vi "Client.vi"() -> ()   [LabVIEW 2021]
uses:
  <vilib>/Utility/miscctls.llb/LVPositionTypeDef.ctl
  MessageType.ctl
panel:
  in  "Server IP Address":string="localhost"
  in  "Stop":bool
  in  "State Change":bool=TRUE
  out "Status":string
  out "GS":enum16{"Player 1 shoot", "Player 2 Shoot"}(ring)
  out "Player 2 Score":u8
  out "Player 1 Score":u8
  in  "Goal Post":cluster{"left":i16, "Size":i16}={"left"=110, "Size"=125}
  out "Goal Post":T1={"left"=110, "top"=0, "right"=235, "bottom"=15}
  out "Box":T1={"left"=139, "top"=147, "right"=181, "bottom"=180}
  out "goal?":bool=TRUE
  out "Del GK":dbl
  out "Defend":bool
  in  "GK":cluster{"horizontal":dbl, "vertical":dbl}={"horizontal"=175.0, "vertical"=20.0}
  in  "Box Size":cluster{"horizontal":dbl, "Vertical":dbl}={"horizontal"=21.0, "Vertical"=33.0}
  in  "Reset":bool
  out "del x":dbl=-0.26666666666666666
  in  "wait":u32=10
  in  "shot?":bool
  in  "Power":dbl(slide)=1.4141414141414141 scale=0.0..10.0
  in  "Ball Size":i16=9
  in  "Ball":cluster{"horizontal":dbl, "vertical":dbl}={"horizontal"=160.0, "vertical"=180.0}
  in  "Shoot":bool
  out "Ground":picture
  # "PLAYER 2"
  # "Misc. Controls"
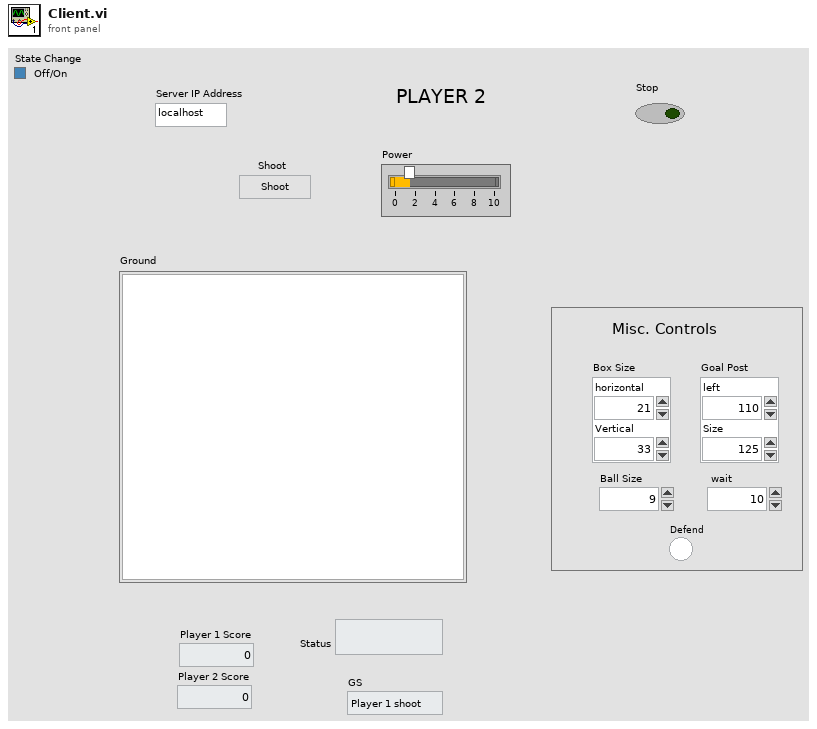
[diagram p1: front panel]
types:
  T1 = cluster{"left":i16, "top":i16, "right":i16, "bottom":i16}
  T2 = typedef "MessageType.ctl" = enum16{"Shoot", "Defend", "Reset", "Score"}
  T3 = typedef "LVPositionTypeDef.ctl" = cluster{"Left":i32, "Top":i32}
  T4 = typedef "LVPoint32TypeDef.ctl" = cluster{"Horizontal":i32, "Vertical":i32}
  T5 = typedef "eventsource.ctl" = u32
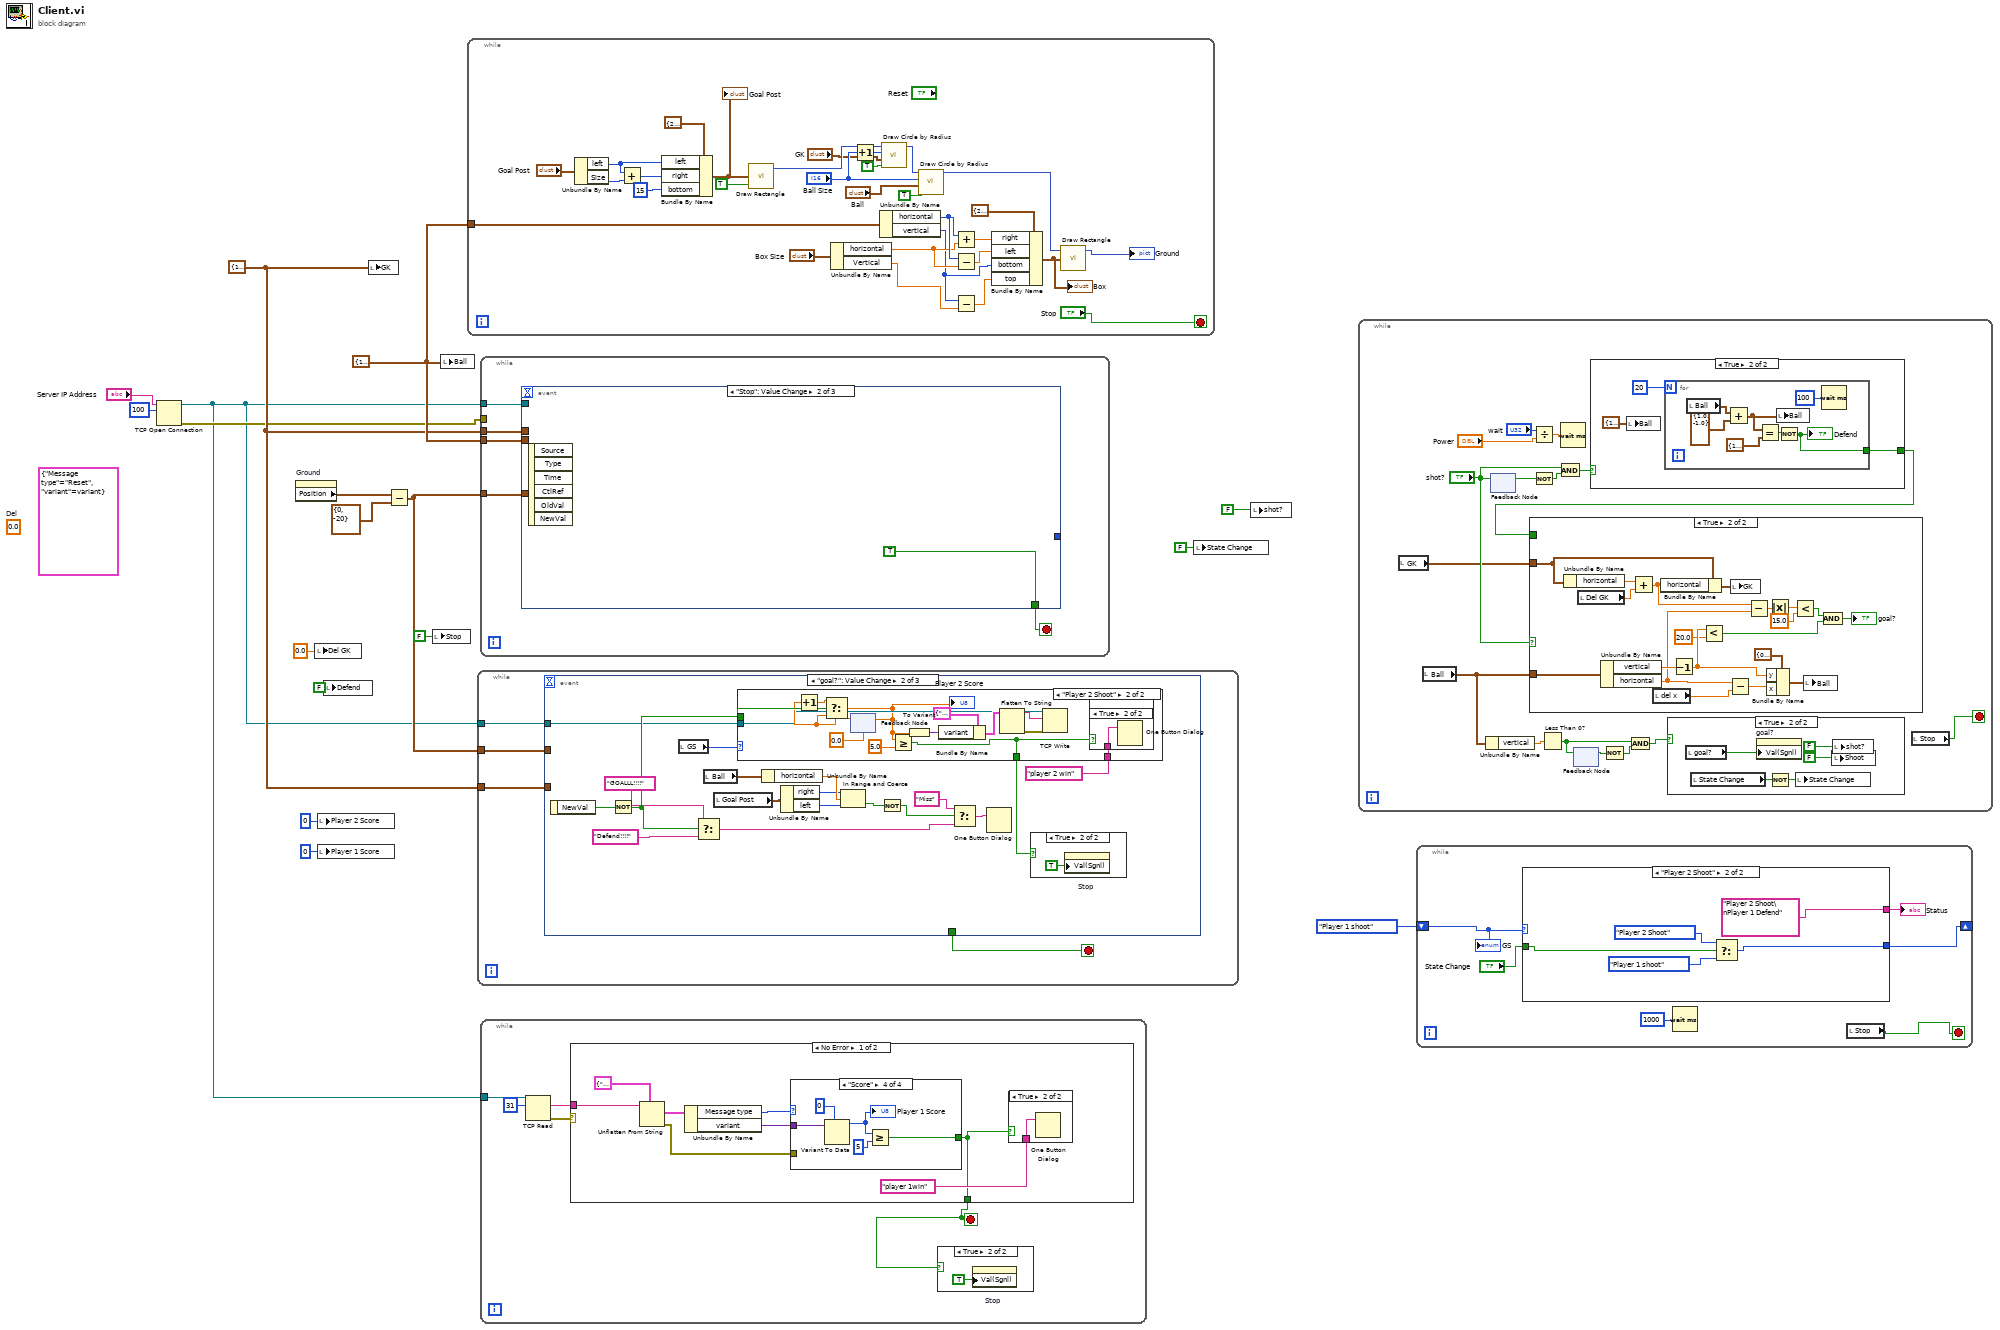
[diagram p0: block diagram]
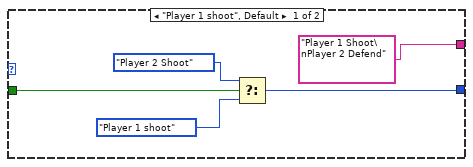
[diagram p2: hidden frame]
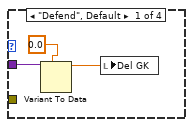
[diagram p5: hidden frame]
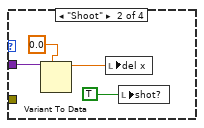
[diagram p6: hidden frame]
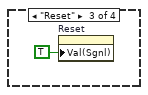
[diagram p7: hidden frame]
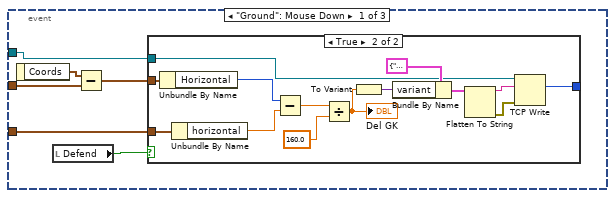
[diagram p9: hidden frame]
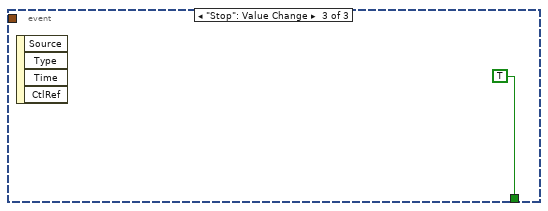
[diagram p14: hidden frame]
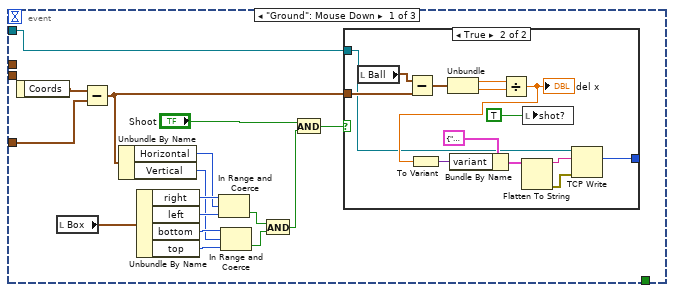
[diagram p18: hidden frame]
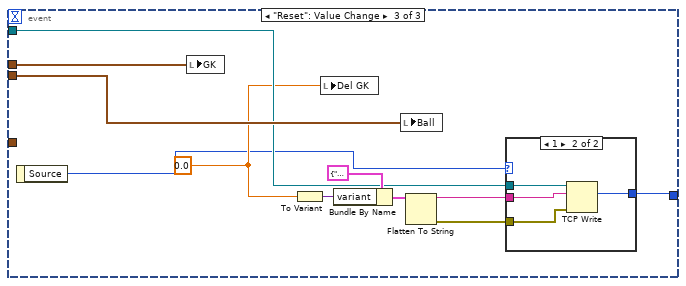
[diagram p20: hidden frame]
diagram:
  (unwired) 0.0  # Del
  (unwired) cluster{"Message type":T2, "variant":variant} {"Message type"=enum."Reset", "variant"=variant}
  w11 = cluster{"horizontal":dbl, "vertical":dbl} {"horizontal"=175.0, "vertical"=20.0} ("GK")
  w14 = cluster{"horizontal":i16, "vertical":i16} {"horizontal"=160, "vertical"=180} ("Ball")
  n1 = TCP Open Connection(address="Server IP Address", remote port or service name=u16 100 ("port")) -> (connection ID=w7:refnum<k5>, error out=w8:errorcluster)  [unwired: 3 in]
  n2 = property on="Ground" class="Pict"() -> ("Position"=w16:T3)  [unwired: 2 in, 2 out]
  n3 = local write "Del GK"(0.0 ("Del GK")) -> ()
  n4 = local write "Player 2 Score"(u8 0 ("Player 2 Score")) -> ()
  n5 = local write "Player 1 Score"(u8 0 ("Player 1 Score")) -> ()
  n6 = local write "Defend"(FALSE ("def")) -> ()
  n7 = local write "GK"(w11) -> ()
  n8 = Subtract(x=w16, y=T3 {"Left"=0, "Top"=-20}) -> (x-y=w13:T3)
  n9 = local write "Stop"(FALSE ("Stop")) -> ()
  n10 = local write "Ball"(w14) -> ()
  n11 = while {
    tunnel: w14 -> [w28]
    stop <- "Stop" stop-if-true
    n12 = Unbundle By Name("Goal Post") -> ("left"=w20:i16, "Size"=w19:i16)
    n13 = Add(x=w20, y=w19) -> (x+y=w43:i16)
    n14 = Bundle By Name(cluster=T1 {"left"=22, "top"=0, "right"=10, "bottom"=10} ("rect"), "left"=w20, "right"=w43, "bottom"=i16 15) -> (w44:T1)
    "Goal Post" <- w44
    n15 = call <vilib>:"Draw Rectangle.vi"("rect"=w44, "fill?(F)"=TRUE) -> ("new picture"=w25:picture)  [unwired: 7 in]
    n16 = Unbundle By Name("Box Size") -> ("horizontal"=w36:dbl, "Vertical"=w33:dbl)
    n17 = Increment(x="Ball Size") -> (x+1=w22:i16)
    n18 = Unbundle By Name(w28) -> ("horizontal"=w37:i16, "vertical"=w35:i16)
    n19 = call <vilib>:"Draw Circle by Radius.vi"("fill?(F)"=TRUE, "pixel center"="GK", "radius"=w22, "picture"=w25) -> ("new picture"=w23:picture)  [unwired: 7 in]
    n20 = call <vilib>:"Draw Circle by Radius.vi"("fill?(F)"=TRUE, "pixel center"="Ball", "radius"="Ball Size", "picture"=w23) -> ("new picture"=w30:picture)  [unwired: 7 in]
    n21 = Add(x=w37, y=w36) -> (x+y=w38:dbl)
    n22 = Subtract(x=w37, y=w36) -> (x-y=w34:dbl)
    n23 = Subtract(x=w35, y=w33) -> (x-y=w32:dbl)
    n24 = Bundle By Name(cluster=T1 {"left"=22, "top"=0, "right"=10, "bottom"=10} ("rect"), "right"=w38, "left"=w34, "bottom"=w35, "top"=w32) -> (w31:T1)
    "Box" <- w31
    n25 = call <vilib>:"Draw Rectangle.vi"("picture"=w30, "rect"=w31) -> ("new picture"=→"Ground":picture)  [unwired: 7 in]
  }
  n26 = while {
    tunnel: w13 -> [w51]
    tunnel: w11 -> [w50]
    tunnel: w7 -> [w49]
    stop <- w48 stop-if-true
    n27 = event shown="[1] \"goal?\": Value Change" {
      selector: _ -> [_ _ _]
      dyn-events: _ -> [_ _ _]
      timeout: _ -> [_ _ _]
      tunnel: w51 -> [w56 _ _]
      tunnel: w50 -> [w54 _ _]
      tunnel: w49 -> [w52 w75 _]
      tunnel: [_ _ TRUE] -> w48
      event "Ground": Mouse Down {
        n28 = event-data() -> ("Coords"=w57:T4)  [unwired: 1 in]
        n29 = local read "Defend"() -> (w53:bool)
        n30 = Subtract(x=w57, y=w56) -> (x-y=w55:T4)
        n31 = case shown="True" w53 {
          tunnel: w55 -> [_ w71]
          tunnel: w54 -> [_ w70]
          tunnel: w52 -> [_ w60]
          tunnel: [_ w58] -> _
          frame False {
          }
          frame True {
            n32 = Unbundle By Name(w71) -> ("Horizontal"=w69:i32)
            n33 = Unbundle By Name(w70) -> ("horizontal"=w68:dbl)
            n34 = Subtract(x=w69, y=w68) -> (x-y=w67:dbl)
            n35 = Divide(x=w67, y=160.0) -> (x/y=w59:dbl)
            "Del GK" <- w59
            n36 = To Variant(anything=w59) -> (Variant=w64:variant)
            n37 = Bundle By Name(cluster=cluster{"Message type":T2, "variant":variant} {"Message type"=enum."Defend", "variant"=variant}, "variant"=w64) -> (w63:cluster{"Message type":T2, "variant":variant})
            n38 = Flatten To String(anything=w63) -> (data string=w61:string, error out=w62:errorcluster)  [unwired: 3 in, 1 out]
            n39 = TCP Write(connection ID=w60, data in=w61, error in (no error)=w62) -> (bytes written=w58:i32)  [unwired: 1 in, 2 out]
          }
        }
      }
      event "goal?": Value Change {
        n40 = event-data() -> ("NewVal"=w89:bool)  [unwired: 1 in]
        n41 = Not(x=w89) -> (.not. x?=w76:bool)
        n42 = local read "GS"() -> (w74:enum16{"Player 1 shoot", "Player 2 Shoot"})
        n43 = Select(t="GOALLL!!!!", s=w76, f="Defend!!!!") -> (s? t:f=w78:string)
        n44 = local read "Ball"() -> (w82:cluster{"horizontal":dbl, "vertical":dbl})
        n45 = local read "Goal Post"() -> (w83:T1)
        n46 = case shown="\"Player 2 Shoot\"" w74 {
          tunnel: w76 -> [_ w99]
          tunnel: w75 -> [_ w96]
          tunnel: "player 2 win" -> [_ w94]
          tunnel: [_ w91] -> w72
          frame "Player 1 shoot", Default {
          }
          frame "Player 2 Shoot" {
            n47 = feedback #1(0.0) -> (w97:dbl)
            n48 = Increment(x=w97) -> (x+1=w98:dbl)
            n49 = Select(t=w98, s=w99, f=w97) -> (s? t:f=w93:dbl)
            "Player 2 Score" <- w93
            n50 = feedback-in #1(w93) -> ()
            n51 = Greater Or Equal?(x=w93, y=5.0) -> (x >= y?=w91:bool)
            n52 = To Variant(anything=w93) -> (Variant=w103:variant)
            n53 = Bundle By Name(cluster=cluster{"Message type":T2, "variant":variant} {"Message type"=enum."Score", "variant"=variant}, "variant"=w103) -> (w102:cluster{"Message type":T2, "variant":variant})
            n54 = Flatten To String(anything=w102) -> (data string=w100:string, error out=w101:errorcluster)  [unwired: 3 in, 1 out]
            n55 = TCP Write(connection ID=w96, data in=w100, error in (no error)=w101) -> ()  [unwired: 1 in, 3 out]
            n56 = case shown="True" w91 {
              tunnel: w94 -> [_ w105]
              frame False {
              }
              frame True {
                n57 = One Button Dialog(message=w105) -> ()  [unwired: 1 in, 1 out]
              }
            }
          }
        }
        n58 = Unbundle By Name(w82) -> ("horizontal"=w86:dbl)
        n59 = Unbundle By Name(w83) -> ("right"=w84:i16, "left"=w85:i16)
        n60 = In Range and Coerce(upper limit=w84, x=w86, lower limit=w85) -> (In Range?=w81:bool)  [unwired: 1 out]
        n61 = Not(x=w81) -> (.not. x?=w77:bool)
        n62 = Select(t="Miss", s=w77, f=w78) -> (s? t:f=w79:string)
        n63 = One Button Dialog(message=w79) -> ()  [unwired: 1 in, 1 out]
        n64 = case shown="True" w72 {
          frame False {
          }
          frame True {
            n65 = property on="Stop" class="Bool (strict)"("Val(Sgnl)"=TRUE ("Value (Signaling)")) -> ()  [unwired: 2 in, 2 out]
          }
        }
      }
      event "Stop": Value Change {
        n66 = event-data() -> ()  [unwired: 1 in, 4 out]
      }
    }
  }
  n67 = while {
    tunnel: w13 -> [w111]
    tunnel: w14 -> [w110]
    tunnel: w11 -> [w109]
    tunnel: w7 -> [w108]
    tunnel: w8 -> [_]
    stop <- w107 stop-if-true
    n68 = event shown="[1] \"Stop\": Value Change" {
      selector: _ -> [_ _ _]
      dyn-events: _ -> [_ _ _]
      timeout: _ -> [_ _ _]
      tunnel: w111 -> [w125 _ _]
      tunnel: w110 -> [_ _ w153]
      tunnel: w109 -> [_ _ w152]
      tunnel: w108 -> [w113 _ w146]
      tunnel: [_ _ w144] -> _
      tunnel: [_ TRUE _] -> w107
      event "Ground": Mouse Down {
        n69 = event-data() -> ("Coords"=w126:T4)  [unwired: 1 in]
        n70 = local read "Box"() -> (w124:T1)
        n71 = Subtract(x=w126, y=w125) -> (x-y=w119:T4)
        n72 = Unbundle By Name(w119) -> ("Horizontal"=w118:i32, "Vertical"=w117:i32)
        n73 = Unbundle By Name(w124) -> ("right"=w123:i16, "left"=w122:i16, "bottom"=w121:i16, "top"=w120:i16)
        n74 = In Range and Coerce(upper limit=w123, x=w118, lower limit=w122) -> (In Range?=w115:bool)  [unwired: 1 out]
        n75 = In Range and Coerce(upper limit=w121, x=w117, lower limit=w120) -> (In Range?=w116:bool)  [unwired: 1 out]
        n76 = And(x=w115, y=w116) -> (x .and. y?=w112:bool)
        n77 = And(x="Shoot", y=w112) -> (x .and. y?=w114:bool)
        n78 = case shown="True" w114 {
          tunnel: w119 -> [_ w140]
          tunnel: w113 -> [_ w129]
          tunnel: [_ w128] -> _
          frame False {
          }
          frame True {
            n79 = local read "Ball"() -> (w139:cluster{"horizontal":dbl, "vertical":dbl})
            n80 = Subtract(x=w139, y=w140) -> (x-y=w138:cluster{dbl, dbl})
            n81 = Unbundle(w138) -> (w137:dbl, w136:dbl)
            n82 = Divide(x=w137, y=w136) -> (x/y=w134:dbl)
            "del x" <- w134
            n83 = To Variant(anything=w134) -> (Variant=w133:variant)
            n84 = Bundle By Name(cluster=cluster{"Message type":T2, "variant":variant} {"Message type"=enum."Shoot", "variant"=variant}, "variant"=w133) -> (w132:cluster{"Message type":T2, "variant":variant})
            n85 = Flatten To String(anything=w132) -> (data string=w130:string, error out=w131:errorcluster)  [unwired: 3 in, 1 out]
            n86 = local write "shot?"(TRUE ("Checkbox")) -> ()
            n87 = TCP Write(connection ID=w129, data in=w130, error in (no error)=w131) -> (bytes written=w128:i32)  [unwired: 1 in, 2 out]
          }
        }
      }
      event "Stop": Value Change {
        n88 = event-data() -> ()  [unwired: 1 in, 6 out]
      }
      event "Reset": Value Change {
        w145 = 0.0 ("Del GK")
        n89 = event-data() -> ("Source"=w143:T5)  [unwired: 1 in]
        n90 = local write "GK"(w152) -> ()
        n91 = To Variant(anything=w145) -> (Variant=w150:variant)
        n92 = local write "Del GK"(w145) -> ()
        n93 = Bundle By Name(cluster=cluster{"Message type":T2, "variant":variant} {"Message type"=enum."Reset", "variant"=variant}, "variant"=w150) -> (w149:cluster{"Message type":T2, "variant":variant})
        n94 = local write "Ball"(w153) -> ()
        n95 = Flatten To String(anything=w149) -> (data string=w147:string, error out=w148:errorcluster)  [unwired: 3 in, 1 out]
        n96 = case shown="1" w143 {
          tunnel: w148 -> [_ w157]
          tunnel: w147 -> [_ w156]
          tunnel: w146 -> [_ w155]
          tunnel: [_ w154] -> w144
          frame 0, Default {
          }
          frame 1 {
            n97 = TCP Write(connection ID=w155, data in=w156, error in (no error)=w157) -> (bytes written=w154:i32)  [unwired: 1 in, 2 out]
          }
        }
      }
    }
  }
  n98 = while {
    tunnel: w7 -> [w162]
    stop <- w158 stop-if-true
    n99 = TCP Read(connection ID=w162, bytes to read=31) -> (data out=w159:string, error out=w160:errorcluster)  [unwired: 3 in, 1 out]
    n100 = case shown="No Error" w160 {
      tunnel: w159 -> [w171 _]
      tunnel: [w164 _] -> w158
      frame No Error {
        n101 = Unflatten From String(type=cluster{"Message type":T2, "variant":variant} {"Message type"=enum."Defend", "variant"=variant}, binary string=w171) -> (value=w169:cluster{"Message type":T2, "variant":variant}, error out=w166:errorcluster)  [unwired: 3 in, 1 out]
        n102 = Unbundle By Name(w169) -> ("Message type"=w168:T2, "variant"=w167:variant)
        n103 = case shown="\"Score\"" w168 {
          tunnel: w167 -> [w175 w179 _ w184]
          tunnel: w166 -> [_ _ _ _]
          tunnel: [_ _ _ w181] -> w164
          frame "Defend", Default {
            n104 = Variant To Data(type=0.0 ("x/y"), Variant=w175) -> (data=w173:dbl)  [unwired: 1 in, 1 out]
            n105 = local write "Del GK"(w173) -> ()
          }
          frame "Shoot" {
            n106 = Variant To Data(type=0.0 ("x/y"), Variant=w179) -> (data=w177:dbl)  [unwired: 1 in, 1 out]
            n107 = local write "del x"(w177) -> ()
            n108 = local write "shot?"(TRUE ("Checkbox")) -> ()
          }
          frame "Reset" {
            n109 = property on="Reset" class="Bool (strict)"("Val(Sgnl)"=TRUE ("Value (Signaling)")) -> ()  [unwired: 2 in, 2 out]
          }
          frame "Score" {
            n110 = Variant To Data(type=u8 0 ("x/y"), Variant=w184) -> (data=w183:u8)  [unwired: 1 in, 1 out]
            "Player 1 Score" <- w183
            n111 = Greater Or Equal?(x=w183, y=u8 5) -> (x >= y?=w181:bool)
          }
        }
        n112 = case shown="True" w164 {
          tunnel: "player 1win" -> [_ w172]
          frame False {
          }
          frame True {
            n113 = One Button Dialog(message=w172) -> ()  [unwired: 1 in, 1 out]
          }
        }
      }
      frame Error {
      }
    }
    n114 = case shown="True" w158 {
      frame False {
      }
      frame True {
        n115 = property on="Stop" class="Bool (strict)"("Val(Sgnl)"=TRUE ("Value (Signaling)")) -> ()  [unwired: 2 in, 2 out]
      }
    }
  }
  n116 = local write "State Change"(FALSE ("State Change")) -> ()
  n117 = local write "shot?"(FALSE ("Checkbox")) -> ()
  n118 = while {
    stop <- w186 stop-if-true
    n119 = local read "GK"() -> (w192:cluster{"horizontal":dbl, "vertical":dbl})
    n120 = local read "Ball"() -> (w198:cluster{"horizontal":dbl, "vertical":dbl})
    n121 = Unbundle By Name(w198) -> ("vertical"=w197:dbl)
    n122 = feedback-in #2("shot?") -> ()
    n123 = feedback #2() -> (w196:bool)  [unwired: 1 in]
    n124 = Not(x=w196) -> (.not. x?=w194:bool)
    n125 = Divide(x="wait", y="Power") -> (x/y=w200:dbl)
    n126 = Less Than 0?(x=w197) -> (x < 0?=w191:bool)
    n127 = And(x="shot?", y=w194) -> (x .and. y?=w193:bool)
    n128 = Wait (ms)(milliseconds to wait=w200) -> ()  [unwired: 1 out]
    n129 = feedback #3() -> (w189:bool)  [unwired: 1 in]
    n130 = feedback-in #3(w191) -> ()
    n131 = case shown="True" w193 {
      tunnel: [_ w202] -> w187
      frame False {
      }
      frame True {
        n132 = local write "Ball"(cluster{"horizontal":i16, "vertical":i16} {"horizontal"=140, "vertical"=200} ("Ball")) -> ()
        n133 = for {
          N: 20 -> [_]
          tunnel: [w205] -> w202
          n134 = local read "Ball"() -> (w211:cluster{"horizontal":dbl, "vertical":dbl})
          n135 = Add(x=w211, y=cluster{"horizontal":dbl, "vertical":dbl} {"horizontal"=1.0, "vertical"=-1.0}) -> (x+y=w208:cluster{"horizontal":dbl, "vertical":dbl})
          n136 = Equal?(x=w208, y=cluster{"horizontal":i16, "vertical":i16} {"horizontal"=160, "vertical"=180} ("Ball")) -> (x = y?=w207:bool)
          n137 = local write "Ball"(w208) -> ()
          n138 = Not(x=w207) -> (.not. x?=w205:bool)
          "Defend" <- w205
          n139 = Wait (ms)(milliseconds to wait=u32 100) -> ()  [unwired: 1 out]
        }
      }
    }
    n140 = case shown="True" "shot?" {
      tunnel: w198 -> [_ w231]
      tunnel: w192 -> [_ w230]
      tunnel: w187 -> [_ _]
      frame False {
      }
      frame True {
        n141 = Unbundle By Name(w230) -> ("horizontal"=w229:dbl)
        n142 = local read "Del GK"() -> (w228:dbl)
        n143 = Unbundle By Name(w231) -> ("vertical"=w235:dbl, "horizontal"=w223:dbl)
        n144 = Add(x=w229, y=w228) -> (x+y=w224:dbl)
        n145 = local read "del x"() -> (w236:dbl)
        n146 = Bundle By Name(cluster=w230, "horizontal"=w224) -> (w227:cluster{"horizontal":dbl, "vertical":dbl})
        n147 = Decrement(x=w235) -> (x-1=w226:dbl)
        n148 = Less?(x=w226, y=20.0) -> (x < y?=w218:bool)
        n149 = Subtract(x=w223, y=w236) -> (x-y=w233:dbl)
        n150 = local write "GK"(w227) -> ()
        n151 = Subtract(x=w224, y=w223) -> (x-y=w222:dbl)
        n152 = Bundle By Name(cluster=cluster{"x":dbl, "y":dbl} {"x"=0.0, "y"=0.0}, "y"=w226, "x"=w233) -> (w232:cluster{"x":dbl, "y":dbl})
        n153 = Absolute Value(x=w222) -> (abs(x)=w221:dbl)
        n154 = Less?(x=w221, y=15.0) -> (x < y?=w219:bool)
        n155 = local write "Ball"(w232) -> ()
        n156 = And(x=w219, y=w218) -> (x .and. y?=→"goal?":bool)
      }
    }
    n157 = Not(x=w189) -> (.not. x?=w188:bool)
    n158 = And(x=w191, y=w188) -> (x .and. y?=w190:bool)
    n159 = case shown="True" w190 {
      frame False {
      }
      frame True {
        n160 = local read "goal?"() -> (w214:bool)
        n161 = local read "State Change"() -> (w213:bool)
        n162 = property on="goal?" class="Bool (strict)"("Val(Sgnl)"=w214) -> ()  [unwired: 2 in, 2 out]
        n163 = Not(x=w213) -> (.not. x?=w212:bool)
        n164 = local write "State Change"(w212) -> ()
        n165 = local write "Shoot"(FALSE ("Checkbox")) -> ()
        n166 = local write "shot?"(FALSE ("Checkbox")) -> ()
      }
    }
    n167 = local read "Stop"() -> (w186:bool)
  }
  n168 = while {
    shift-right: [w239] -> _
    shift-left: enum16{"Player 1 shoot", "Player 2 Shoot"}."Player 1 shoot" -> [w242]
    stop <- w237 stop-if-true
    n169 = case shown="\"Player 2 Shoot\"" w242 {
      tunnel: ["Player 1 Shoot\nPlayer 2 Defend" "Player 2 Shoot\nPlayer 1 Defend"] -> w241
      tunnel: [w244 w248] -> w239
      tunnel: "State Change" -> [w243 w249]
      frame "Player 1 shoot", Default {
        n170 = Select(t=enum16{"Player 1 shoot", "Player 2 Shoot"}."Player 2 Shoot", s=w243, f=enum16{"Player 1 shoot", "Player 2 Shoot"}."Player 1 shoot") -> (s? t:f=w244:enum16{"Player 1 shoot", "Player 2 Shoot"})
      }
      frame "Player 2 Shoot" {
        n171 = Select(t=enum16{"Player 1 shoot", "Player 2 Shoot"}."Player 2 Shoot", s=w249, f=enum16{"Player 1 shoot", "Player 2 Shoot"}."Player 1 shoot") -> (s? t:f=w248:enum16{"Player 1 shoot", "Player 2 Shoot"})
      }
    }
    "Status" <- w241
    n172 = Wait (ms)(milliseconds to wait=u32 1000) -> ()  [unwired: 1 out]
    n173 = local read "Stop"() -> (w237:bool)
    "GS" <- w242
  }
